vi "SH_calcDistance.vi"(1 "Time series":dbl[](array[numeric]), 3 "Shapelet (normalized)":dbl[](array[numeric])) -> (0 "Distance out":dbl)   [LabVIEW 2016, in "Shapelets Search (Brute Force).lvlib"]
uses:
  Shapelets Search (Brute Force).lvlib
  <vilib>/Analysis/baseanly.llb/Normalize Vector.vi
  <vilib>/Analysis/NI_AALBase.lvlib
panel:
  # "This VI is a part of BCI Design library, http://www.ru-bci.org \nCopyright © 2020, Sotnikov Peter, All rights reserved. License: GNU GPLv3"
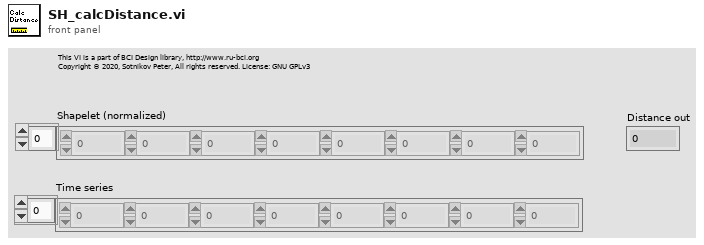
[diagram p1: front panel]
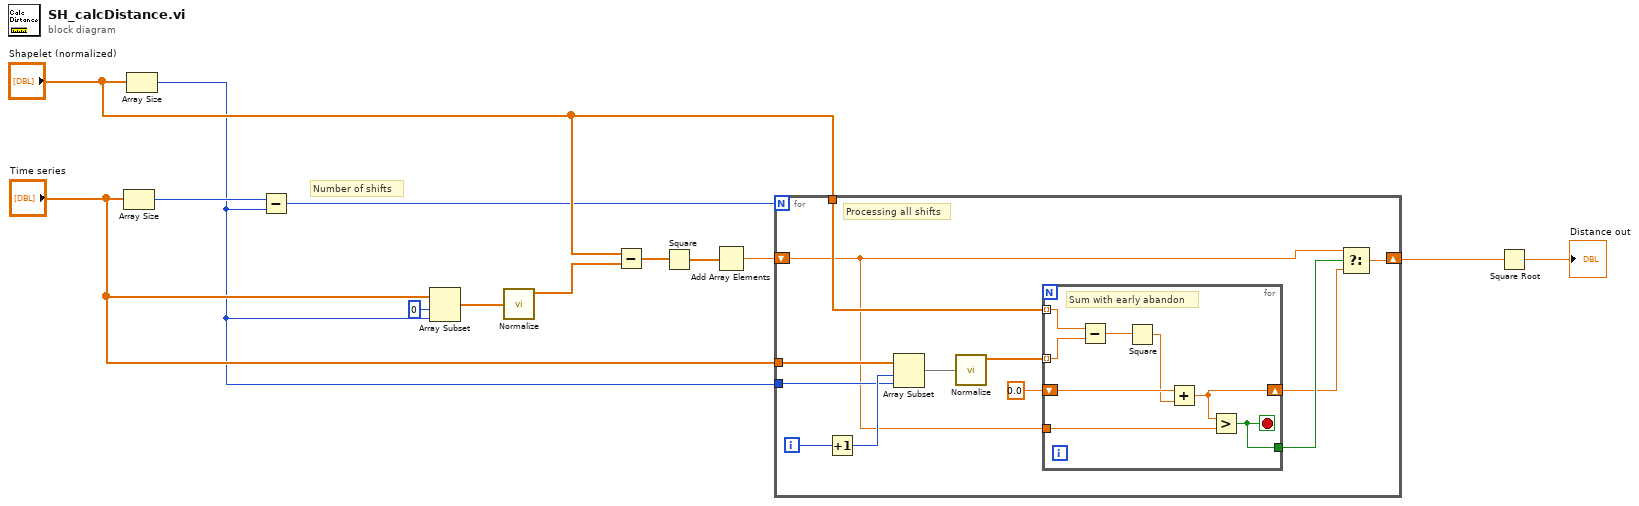
[diagram p0: block diagram]
diagram:
  # "Number of shifts"
  n1 = Array Size(array="Time series") -> (size(s)=w13:i32)
  n2 = Array Size(array="Shapelet (normalized)") -> (size(s)=w3:i32)
  n3 = Subtract(x=w13, y=w3) -> (x-y=w4:i32)
  n4 = Array Subset(array="Time series", index=0, length=w3) -> (w11:dbl[])
  n5 = call-poly <vilib>:"Normalize.vi"("Vector"=w11) -> ("Normalized Vector"=w10:dbl[])  [unwired: 1 in, 3 out]
  n6 = Subtract(x="Shapelet (normalized)", y=w10) -> (x-y=w9:dbl[])
  n7 = Square(x=w9) -> (x^2=w8:dbl[])
  n8 = Add Array Elements(numeric array=w8) -> (sum=w7:dbl)
  n9 = for {
    N: w4 -> [_]
    shift-right: [w17] -> w1
    shift-left: w7 -> [w16]
    tunnel: "Shapelet (normalized)" -> [w20]
    tunnel: "Time series" -> [w25]
    tunnel: w3 -> [w22]
    i -> [w24]
    # "Processing all shifts"
    n10 = Increment(x=w24) -> (x+1=w23:i32)
    n11 = Array Subset(array=w25, index=w23, length=w22) -> (w21:dbl[])
    n12 = call-poly <vilib>:"Normalize.vi"("Vector"=w21) -> ("Normalized Vector"=w19:dbl[])  [unwired: 1 in, 3 out]
    n13 = for {
      tunnel: w20 -> [w32] mode=indexing
      tunnel: w19 -> [w31] mode=indexing
      shift-right: [w28] -> w14
      shift-left: 0.0 -> [w30]
      tunnel: w16 -> [w27]
      tunnel: [w26] -> w15
      stop <- w26 stop-if-true
      # "Sum with early abandon"
      n14 = Subtract(x=w32, y=w31) -> (x-y=w33:dbl)
      n15 = Square(x=w33) -> (x^2=w29:dbl)
      n16 = Add(x=w30, y=w29) -> (x+y=w28:dbl)
      n17 = Greater?(x=w28, y=w27) -> (0:w26:bool)
    }
    n18 = Select(t=w16, s=w15, f=w14) -> (s? t:f=w17:dbl)
  }
  n19 = Square Root(x=w1) -> (sqrt(x)=→"Distance out":dbl)
